vi "parseEnumerationFromModule.vi"(8 "error in (no error)":errorcluster, 11 "Module in":refnum<class "Module.lvclass">) -> (0 "error out":errorcluster, 3 "Module out":refnum<class "Module.lvclass">)   [LabVIEW 2016, in "Module.lvclass"]
uses:
  Module.lvclass
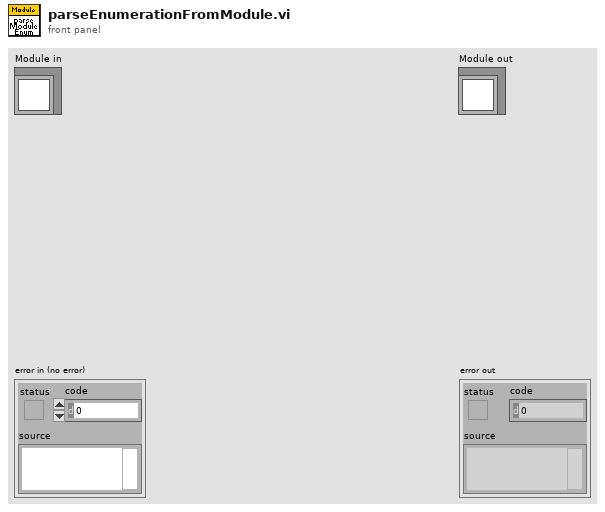
[diagram p1: front panel]
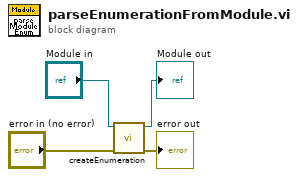
[diagram p0: block diagram]
diagram:
  n1 = call "createEnumeration.vi"("error in (no error)"="error in (no error)", "Module in"="Module in") -> ("error out"=→"error out":errorcluster, "Module out"=→"Module out":refnum<class "Module.lvclass">)  [unwired: 8 in]
